vi "sync_read_write.vi"() -> ()   [LabVIEW 2015]
uses:
  dxl_x86_c.lvlib/dxl_x86_c.lvlib
panel:
  out "groupread_num":i32
  in  "LEN_PRO_\nPRESENT_POSITION":u16=4
  out "groupwrite_num":i32
  in  "LEN_PRO_\nGOAL_POSITION":u16=4
  out "value : PRO (knob)\npresent position 2":i32(knob) scale=150000.0..-150000.0
  in  "dynamixe2_id":u8=2
  in  "device_name":string="COM8"
  in  "ADDR_PRO_\nPRESENT_POSITION":u16=611
  in  "ADDR_PRO_\nGOAL_POSITION":u16=596
  in  "ADDR_PRO_\nTORQUE_ENABLE":u16=562
  out "protocol_version":dbl=2.0
  out "value : PRO (knob)\npresent position 1":i32(knob) scale=150000.0..-150000.0
  in  "terminate":bool
  out "port_num":i32
  in  "value : PRO (dial)\ngoal position":i32(knob) scale=150000.0..-150000.0
  in  "dynamixel1_id":u8=1
  in  "baud_rate":i32=1000000
  # "sync_write.vi\n\nCreated on: 2016. 6. 8\nAuthor: Leon Ryu Woon Jung\n\n*********     Read and Write Example      *********\n\n\nAvailable DXL model on this example : All models using Protocol 1.0\nThis example is designed for using two Dynamixel MX-28, and an USB2DYNAMIXEL.\nTo use another Dynamixel model, such as X series, see their details in E-Manual(support.robotis.com) \n   and edit \"numeric control\"s seen left with \"Edit Text\" tool.\nBe sure that Dynamixel MX properties are already set as %% ID : 1 / Baudnum : 1 (Baudrate : 1000000 [1M])\n\n1. Run example by click above \"Run\" button (below \"Edit\" menu).\n2. Drag \"dial\" then you may see the Dynamixel and \"knob\"s rotating\n3. To finish the example, press \"terminate\" button."
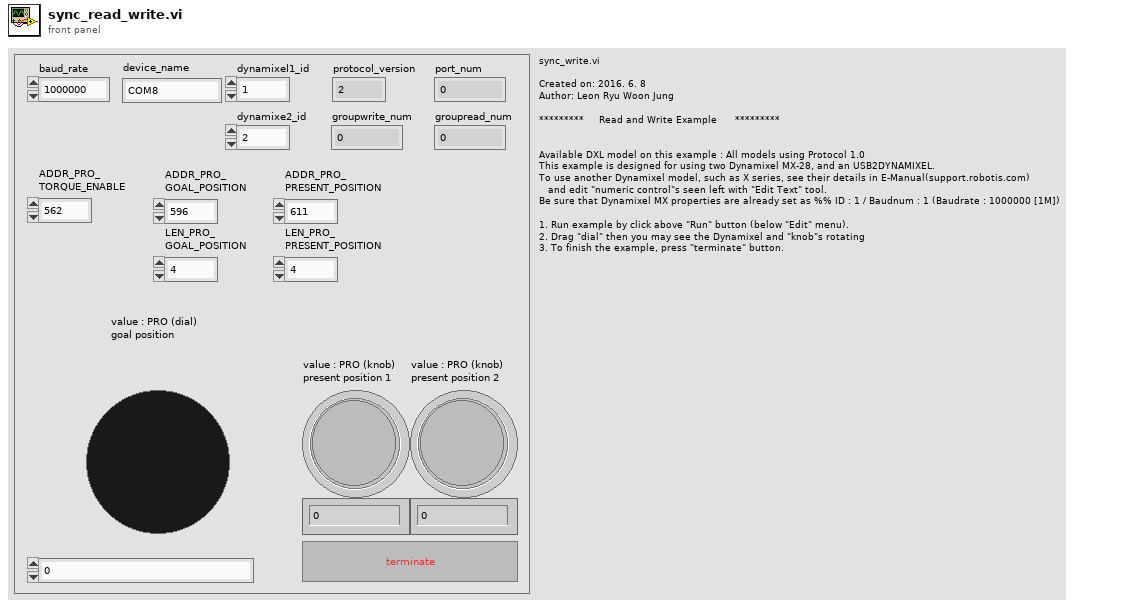
[diagram p1: front panel]
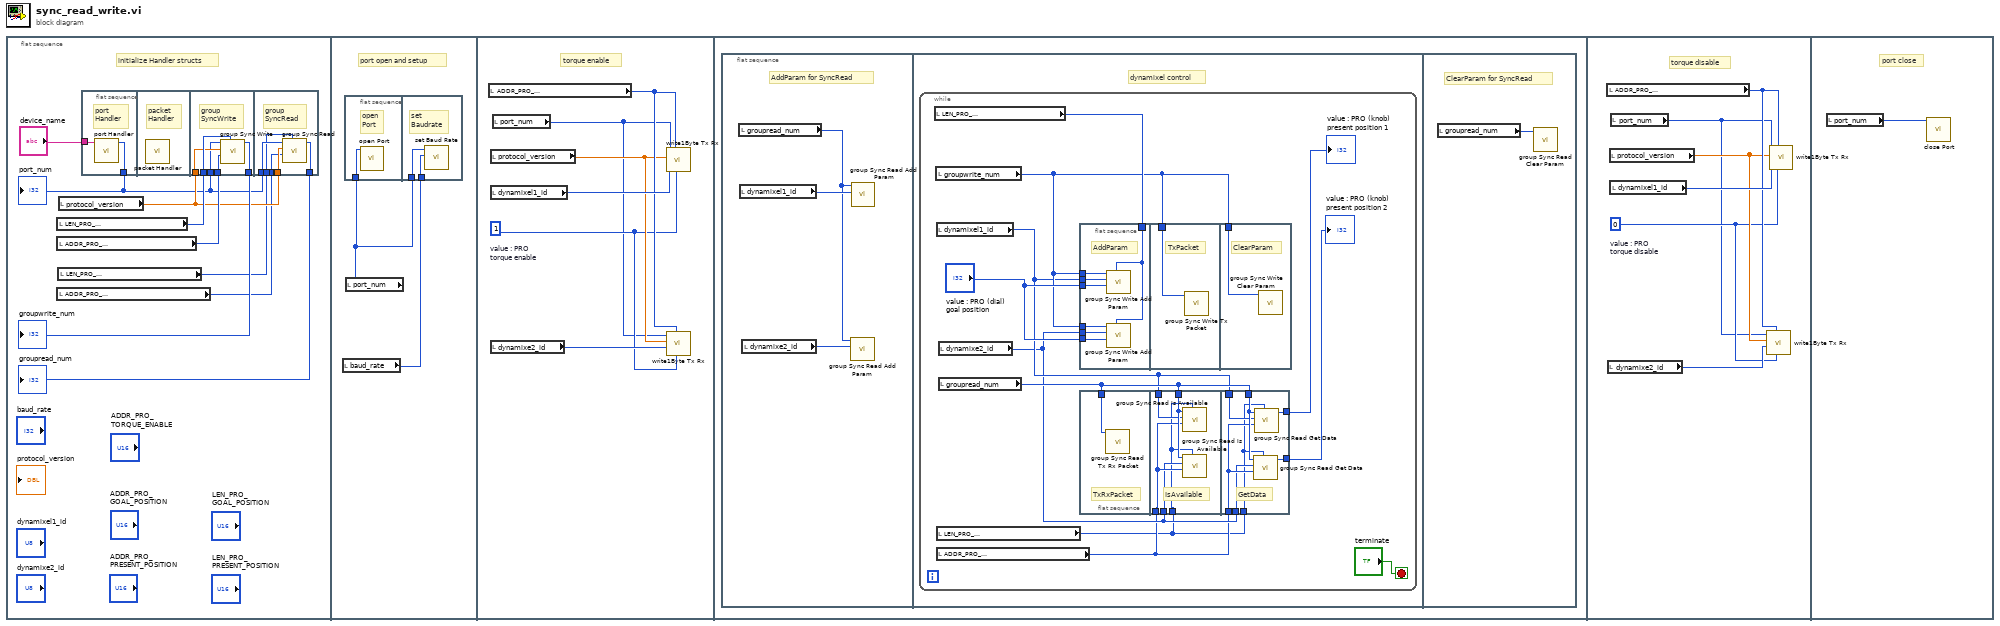
[diagram p0: block diagram]
diagram:
  n1 = flat-sequence {
    frame #0 {
      # "initialize Handler structs"
      n2 = local read "LEN_PRO_\nGOAL_POSITION"() -> (w8:u16)
      n3 = local read "ADDR_PRO_\nGOAL_POSITION"() -> (w7:u16)
      n4 = local read "ADDR_PRO_\nPRESENT_POSITION"() -> (w3:u16)
      n5 = local read "LEN_PRO_\nPRESENT_POSITION"() -> (w1:u16)
      n6 = local read "protocol_version"() -> (w4:dbl)
      n7 = flat-sequence {
        tunnel: "device_name" -> [w11]
        tunnel: [w10] -> w2
        tunnel: w8 -> [w16]
        tunnel: w7 -> [w15]
        tunnel: w4 -> [w14]
        tunnel: w2 -> [w13]
        tunnel: [w12] -> w6
        tunnel: [w21] -> w5
        tunnel: w4 -> [w20]
        tunnel: w3 -> [w19]
        tunnel: w2 -> [w18]
        tunnel: w1 -> [w17]
        frame #0 {
          # "port\nHandler"
          n8 = call "port Handler.vi"("port_name"=w11) -> ("function return"=w10:i32)  [unwired: 10 in]
        }
        frame #1 {
          # "packet\nHandler"
          n9 = call "packet Handler.vi"() -> ()  [unwired: 12 in]
        }
        frame #2 {
          # "group\nSyncWrite"
          n10 = call "group Sync Write.vi"("data_length"=w16, "start_address"=w15, "protocol_version"=w14, "port_num"=w13) -> ("function return"=w12:i32)  [unwired: 7 in]
        }
        frame #3 {
          # "group\nSyncRead"
          n11 = call "group Sync Read.vi"("data_length"=w17, "start_address"=w19, "protocol_version"=w20, "port_num"=w18) -> ("function return"=w21:i32)  [unwired: 7 in]
        }
      }
      "port_num" <- w2
      "groupwrite_num" <- w6
      "groupread_num" <- w5
    }
    frame #1 {
      # "port open and setup"
      n12 = local read "baud_rate"() -> (w22:i32)
      n13 = flat-sequence {
        tunnel: w23 -> [w24]
        tunnel: w23 -> [w26]
        tunnel: w22 -> [w25]
        frame #0 {
          # "open\nPort"
          n14 = call "open Port.vi"("port_num"=w24) -> ()  [unwired: 10 in, 1 out]
        }
        frame #1 {
          # "set\nBaudrate"
          n15 = call "set Baud Rate.vi"("baudrate"=w25, "port_num"=w26) -> ()  [unwired: 9 in, 1 out]
        }
      }
      n16 = local read "port_num"() -> (w23:i32)
    }
    frame #2 {
      w28 = 1  # value : PRO torque enable
      # "torque enable"
      n17 = local read "ADDR_PRO_\nTORQUE_ENABLE"() -> (w31:u16)
      n18 = local read "protocol_version"() -> (w30:dbl)
      n19 = local read "dynamixel1_id"() -> (w32:u8)
      n20 = local read "dynamixe2_id"() -> (w29:u8)
      n21 = local read "port_num"() -> (w27:i32)
      n22 = call "write1Byte Tx Rx.vi"("data"=w28, "address"=w31, "id"=w32, "protocol_version"=w30, "port_num"=w27) -> ()  [unwired: 7 in]
      n23 = call "write1Byte Tx Rx.vi"("data"=w28, "address"=w31, "id"=w29, "protocol_version"=w30, "port_num"=w27) -> ()  [unwired: 7 in]
    }
    frame #3 {
      n24 = flat-sequence {
        frame #0 {
          # "AddParam for SyncRead"
          n25 = local read "groupread_num"() -> (w33:i32)
          n26 = local read "dynamixel1_id"() -> (w35:u8)
          n27 = local read "dynamixe2_id"() -> (w34:u8)
          n28 = call "group Sync Read Add Param.vi"("id"=w34, "group_num"=w33) -> ()  [unwired: 9 in, 1 out]
          n29 = call "group Sync Read Add Param.vi"("id"=w35, "group_num"=w33) -> ()  [unwired: 9 in, 1 out]
        }
        frame #1 {
          # "dynamixel control"
          n30 = while {
            stop <- "terminate" stop-if-true
            n31 = local read "LEN_PRO_\nGOAL_POSITION"() -> (w45:u16)
            n32 = local read "groupwrite_num"() -> (w43:i32)
            n33 = local read "dynamixel1_id"() -> (w41:u8)
            n34 = local read "LEN_PRO_\nPRESENT_POSITION"() -> (w38:u16)
            n35 = local read "ADDR_PRO_\nPRESENT_POSITION"() -> (w39:u16)
            n36 = local read "dynamixe2_id"() -> (w40:u8)
            n37 = local read "groupread_num"() -> (w42:i32)
            n38 = flat-sequence {
              tunnel: w45 -> [w66]
              tunnel: w43 -> [w65]
              tunnel: w43 -> [w64]
              tunnel: w41 -> [w63]
              tunnel: w40 -> [w62]
              tunnel: "value : PRO (dial)\ngoal position" -> [w61]
              tunnel: "value : PRO (dial)\ngoal position" -> [w60]
              tunnel: w43 -> [w67]
              tunnel: w43 -> [w68]
              frame #0 {
                # "AddParam"
                n39 = call "group Sync Write Add Param.vi"("data_length"=w66, "data"=w60, "id"=w63, "group_num"=w65) -> ()  [unwired: 7 in, 1 out]
                n40 = call "group Sync Write Add Param.vi"("data_length"=w66, "data"=w61, "id"=w62, "group_num"=w64) -> ()  [unwired: 7 in, 1 out]
              }
              frame #1 {
                # "TxPacket"
                n41 = call "group Sync Write Tx Packet.vi"("group_num"=w67) -> ()  [unwired: 11 in]
              }
              frame #2 {
                # "ClearParam"
                n42 = call "group Sync Write Clear Param.vi"("group_num"=w68) -> ()  [unwired: 11 in]
              }
            }
            n43 = flat-sequence {
              tunnel: w42 -> [w47]
              tunnel: w42 -> [w52]
              tunnel: w41 -> [w51]
              tunnel: w40 -> [w49]
              tunnel: w39 -> [w50]
              tunnel: w38 -> [w48]
              tunnel: w42 -> [w59]
              tunnel: w41 -> [w58]
              tunnel: w40 -> [w54]
              tunnel: w39 -> [w55]
              tunnel: w38 -> [w53]
              tunnel: [w57] -> w37
              tunnel: [w56] -> w36
              frame #0 {
                # "TxRxPacket"
                n44 = call "group Sync Read Tx Rx Packet.vi"("group_num"=w47) -> ()  [unwired: 11 in]
              }
              frame #1 {
                # "IsAvailable"
                n45 = call "group Sync Read Is Available.vi"("data_length"=w48, "address"=w50, "id"=w51, "group_num"=w52) -> ()  [unwired: 7 in, 1 out]
                n46 = call "group Sync Read Is Available.vi"("data_length"=w48, "address"=w50, "id"=w49, "group_num"=w52) -> ()  [unwired: 7 in, 1 out]
              }
              frame #2 {
                # "GetData"
                n47 = call "group Sync Read Get Data.vi"("data_length"=w53, "address"=w55, "id"=w54, "group_num"=w59) -> ("function return"=w56:u32)  [unwired: 7 in]
                n48 = call "group Sync Read Get Data.vi"("data_length"=w53, "address"=w55, "id"=w58, "group_num"=w59) -> ("function return"=w57:u32)  [unwired: 7 in]
              }
            }
            "value : PRO (knob)\npresent position 1" <- w37
            "value : PRO (knob)\npresent position 2" <- w36
          }
        }
        frame #2 {
          # "ClearParam for SyncRead"
          n49 = local read "groupread_num"() -> (w69:i32)
          n50 = call "group Sync Read Clear Param.vi"("group_num"=w69) -> ()  [unwired: 11 in]
        }
      }
    }
    frame #4 {
      w71 = 0  # value : PRO torque disable
      # "torque disable"
      n51 = local read "ADDR_PRO_\nTORQUE_ENABLE"() -> (w74:u16)
      n52 = local read "dynamixe2_id"() -> (w72:u8)
      n53 = local read "protocol_version"() -> (w73:dbl)
      n54 = local read "dynamixel1_id"() -> (w75:u8)
      n55 = local read "port_num"() -> (w70:i32)
      n56 = call "write1Byte Tx Rx.vi"("data"=w71, "address"=w74, "id"=w72, "protocol_version"=w73, "port_num"=w70) -> ()  [unwired: 7 in]
      n57 = call "write1Byte Tx Rx.vi"("data"=w71, "address"=w74, "id"=w75, "protocol_version"=w73, "port_num"=w70) -> ()  [unwired: 7 in]
    }
    frame #5 {
      # "port close"
      n58 = local read "port_num"() -> (w76:i32)
      n59 = call "close Port.vi"("port_num"=w76) -> ()  [unwired: 11 in]
    }
  }
